vi "VectorNav-ParseRead.vi"(10 "Input String":string=" 12, 213, 26") -> (2 "Output Array":dbl[](array[numeric]))   [LabVIEW 2010]
uses:
  <vilib>/regexp/Match Regular Expression.xnode
panel:
  # "This VI takes a comma-\ndelimted string input and converts it to an array of strings and an array of numbers."
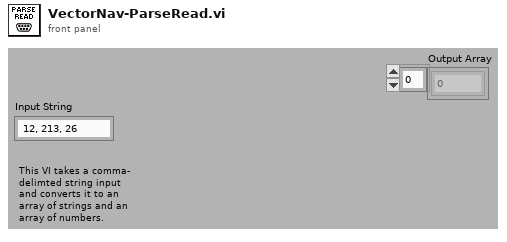
[diagram p1: front panel]
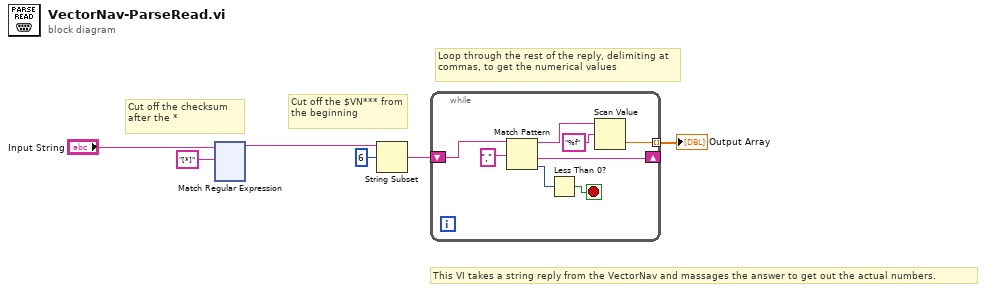
[diagram p0: block diagram]
diagram:
  # "Loop through the rest of the reply, delimiting at commas, to get the numerical values"
  # "Cut off the $VN*** from the beginning"
  # "Cut off the checksum after the *"
  # "This VI takes a string reply from the VectorNav and massages the answer to get out the actual numbers."
  n1 = xnode "Match Regular Expression"("input string"="Input String", "regular expression"="[*]") -> ("before match"=w4:string)  [unwired: 4 in, 4 out]
  n2 = String Subset(string=w4, offset (0)=6) -> (substring=w3:string)  [unwired: 1 in]
  n3 = while {
    shift-right: [w12] -> _
    shift-left: w3 -> [w14]
    tunnel: [w7] -> w1 mode=indexing
    stop <- w10 stop-if-true
    n4 = Match Pattern(string=w14, regular expression=",") -> (before substring=w8:string, after substring=w12:string, offset past match=w11:i32)  [unwired: 2 out]
    n5 = Less Than 0?(x=w11) -> (x < 0?=w10:bool)
    n6 = Scan Value(string=w8, format string="%f") -> (value=w7:dbl)  [unwired: 1 in, 1 out]
  }
  "Output Array" <- w1
